vi "GetControlRefFromControlArray.vi"(0 "Controls[]":refnum<vi>[](array[refnum]), 7 "Control Path":string, 11 "error In":errorcluster) -> (4 "Remaining Controls[]":refnum<vi>[](array[refnum]), 8 "Target Control":refnum<vi>, 15 "error out":errorcluster)   [LabVIEW 2016, in "Drona.lvlib" / "GetControlRef.lvlib"]
doc: "This VI gives the desired control reference from the array of control references"
uses:
  GetControlRef.lvlib
  Drona.lvlib
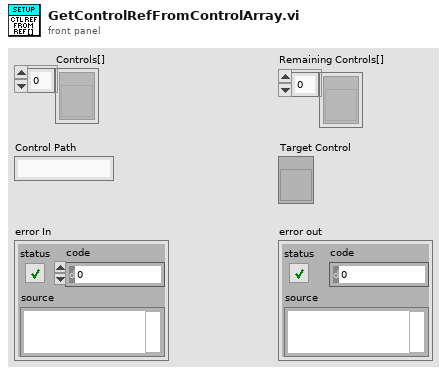
[diagram p1: front panel]
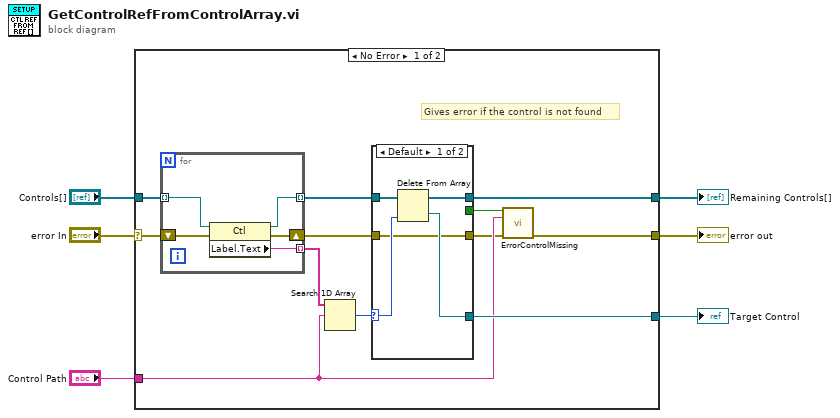
[diagram p0: block diagram]
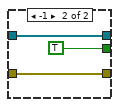
[diagram p2: hidden frame]
diagram:
  n1 = case shown="No Error" "error In" {
    selector: "error In" -> [w15 w33]
    tunnel: "Controls[]" -> [w18 w32]
    tunnel: [w17 w32] -> w5
    tunnel: [w16 _] -> w4
    tunnel: [w14 w33] -> w2
    tunnel: "Control Path" -> [w13 _]
    frame No Error {
      # "Gives error if the control is not found"
      n2 = for {
        tunnel: w18 -> [w31] mode=indexing
        shift-right: [w29] -> w8
        shift-left: w15 -> [w30]
        tunnel: [w28] -> w11 mode=indexing
        tunnel: [w27] -> w12 mode=indexing
        n3 = property class="Ctl"(reference=w31, error in=w30) -> (reference out=w28:refnum<vi>, error out=w29:errorcluster, "Label.Text"=w27:string)
      }
      n4 = Search 1D Array(1D array=w12, element=w13) -> (index of element=w10:i32)  [unwired: 1 in]
      n5 = case shown="Default" w10 {
        selector: w10 -> [w21 _]
        tunnel: [w23 w26] -> w17
        tunnel: w11 -> [w22 w26]
        tunnel: [_ TRUE] -> w9
        tunnel: [w20 _] -> w16
        tunnel: [w19 w24] -> w7
        tunnel: w8 -> [w19 w24]
        frame Default {
          n6 = Delete From Array(array=w22, index=w21) -> (deleted portion=w20:refnum<vi>, array with subset deleted=w23:refnum<vi>[])  [unwired: 1 in]
        }
        frame -1 {
        }
      }
      n7 = call "ErrorControlMissing.vi"("Create Error?"=w9, "Control Name"=w13, "error in"=w7) -> ("error out"=w14:errorcluster)  [unwired: 12 in]
    }
    frame Error {
    }
  }
  "Remaining Controls[]" <- w5
  "Target Control" <- w4
  "error out" <- w2
